vi "Global_Stop_3.vi"() -> ()   [LabVIEW 2020]
panel:
  out "global stop 3":bool
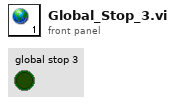
[diagram p1: front panel]
diagram:
